vi "Controller Reference Orbit Selection.vi"(10 "Reference Orbits":dbl[][](array[numeric]), 11 "selected":i32) -> (2 "Selected Reference Orbit":dbl[](array[numeric]))   [LabVIEW 2011, in "Controller VIs.lvlib"]
uses:
  Controller VIs.lvlib
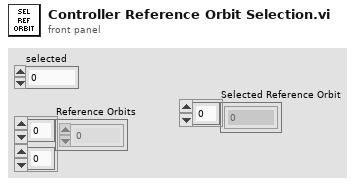
[diagram p1: front panel]
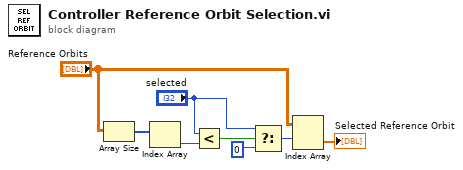
[diagram p0: block diagram]
diagram:
  n1 = Array Size(array="Reference Orbits") -> (size(s)=w4:i32[])
  n2 = Index Array(array=w4) -> (element=w5:i32)  [unwired: 1 in]
  n3 = Less?(x="selected", y=w5) -> (x < y?=w6:bool)
  n4 = Select(t="selected", s=w6, f=0) -> (s? t:f=w3:i32)
  n5 = Index Array(array="Reference Orbits", index (row)=w3) -> (element=→"Selected Reference Orbit":dbl[])  [unwired: 1 in]
